vi "SPI Set CS Logic Level.vi"(8 "Error In":errorcluster, 9 "CS Logic Level":T1, 10 "SPI Channel":u8, 11 "LINX Device Config":T2) -> (0 "Error Out":errorcluster, 3 "LINX Device Config":T2)   [LabVIEW 2013, in "LVH-LINX.lvlib" / "Device.lvlib"]
doc: "Set the chip select logic level (active high or active low) for the specified SPI Channel.\n\n0 - Active Low\n1 - Active High"
uses:
  Device.lvlib
  Type Defs/LINX Device Config.ctl
  Type Defs/Interface.ctl
  Type Defs/TCP Config.ctl
  Type Defs/Device Family.ctl
  Type Defs/Channels.ctl
  Type Defs/Peripherals/SPI/SPI CS Logic Level.ctl
  Type Defs/Error Type.ctl
  LVH-LINX.lvlib
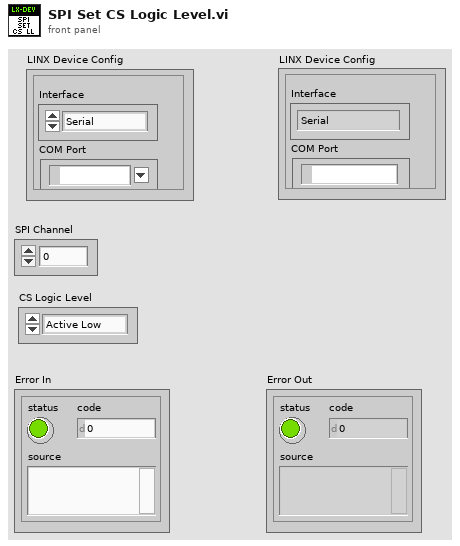
[diagram p1: front panel]
types:
  T1 = typedef "LVH-LINX.lvlib/SPI CS Logic Level.ctl" = enum8{"Active Low", "Active High"}
  T2 = typedef "LVH-LINX.lvlib/Device.lvlib/LINX Device Config.ctl" = cluster{"Interface":T3, "COM Port":refnum<visa-resource-name>, "TCP Configuration":T4, "Device Family":T5, "Device ID":u8, "Device Name":string, "TCP Ref":refnum<k5>, "Channels":T6}
  T3 = typedef "LVH-LINX.lvlib/Interface.ctl" = enum16{"Serial", "TCP"}
  T4 = typedef "LVH-LINX.lvlib/Device.lvlib/TCP Config.ctl" = cluster{"IP Address":string, "Port":u16}
  T5 = typedef "LVH-LINX.lvlib/Device Family.ctl" = enum8{"National Instruments", "Digilent", "Arduino"}
  T6 = typedef "LVH-LINX.lvlib/Channels.ctl" = cluster{"DI Channels":u8[], "DO Channels":u8[], "AI":u8[], "AO":u8[], "PWM":u8[], "QE":u8[], "UART":u8[], "I2C 2":u8[], "SPI":u8[], "CAN":u8[], "AI Ref (V)":dbl, "AO Resolution (Bits)":u8, "AO Ref (V)":dbl}
  T7 = typedef "LVH-LINX.lvlib/Error Type.ctl" = enum16{"Unknown", "Timeout", "Corrupt Return Packet", "Unable To Connect", "Command Not Supported", "Channel DNE", "Invalid COM Config", "Firmware Version Mismatch"}
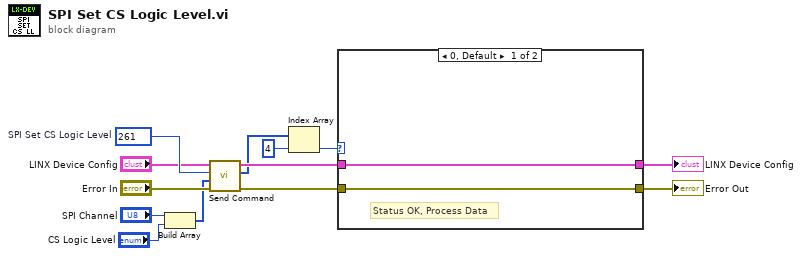
[diagram p0: block diagram]
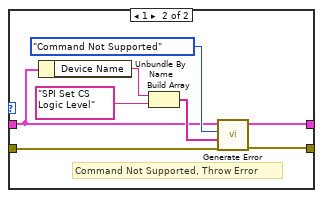
[diagram p2: hidden frame]
diagram:
  w12 = u16 261  # SPI Set CS Logic Level
  n1 = Build Array("SPI Channel", "CS Logic Level") -> (w5:u8[])
  n2 = call "Send Command.vi"("Error In"="Error In", "ARGS"=w5, "CMD"=w12, "LINX Device Config"="LINX Device Config") -> ("Error Out"=w7:errorcluster, "Response"=w4:u8[], "LINX Device Config"=w9:T2)  [unwired: 4 in, 1 out]
  n3 = Index Array(array=w4, index=4) -> (element=w2:u8)
  n4 = case shown="0, Default" w2 {
    tunnel: [w15 w21] -> w10
    tunnel: w9 -> [w15 w17]
    tunnel: [w14 w22] -> w8
    tunnel: w7 -> [w14 w23]
    frame 0, Default {
      # "Status OK, Process Data"
    }
    frame 1 {
      # "Command Not Supported, Throw Error"
      n5 = Unbundle By Name(w17) -> ("Device Name"=w16:string)
      n6 = Build Array(w16, "SPI Set CS Logic Level") -> (w18:string[])
      n7 = call "Generate Error.vi"("Error In"=w23, "Arguments"=w18, "Error Type"=Error_Type."Command Not Supported", "LINX Device Config"=w17) -> ("Error Out"=w22:errorcluster, "LINX Device Config"=w21:T2)  [unwired: 6 in]
    }
  }
  "Error Out" <- w8
  "LINX Device Config" <- w10
